vi "IMAQdx_set_attrib.vi"(4 "error in":errorcluster, 5 "value":variant, 6 "attribute":string, 7 "IMAQdx in":T1) -> (0 "error out":errorcluster, 2 "attrib out":variant, 3 "IMAQdx out":T1)   [LabVIEW 2010]
uses:
  <vilib>/userDefined/High Color/IMAQdx.ctl
  resource/objmgr/imaqdx.rc
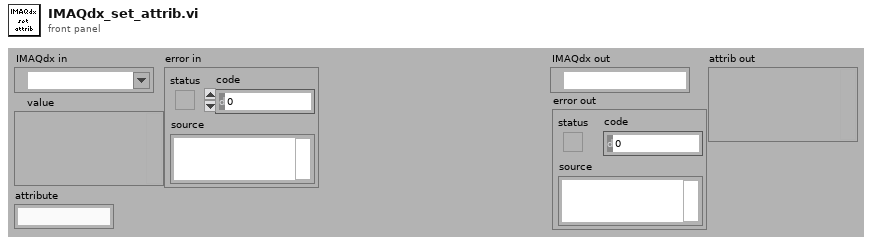
[diagram p1: front panel]
types:
  T1 = typedef "IMAQdx.ctl" = refnum<k21>
  T2 = typedef "Type Descriptor Enumeration__ogtk.ctl" = enum8{"<Null>", "I8", "I16", "I32", "I64", "U8", "U16", "U32", "U64", "SGL", "DBL", "EXT", "CSG", "CDB", "CXT", "0x0F", "0x10", "0x11", "0x12", "0x13", "0x14", "Enum U8", "Enum U16", "Enum U32", "Enum U64", "SGL PQ", "DBL PQ", "EXT PQ", "CSG PQ", "CDB PQ", "CXT PQ", "0x1F", "0x20", "Boolean", "0x22", "0x23", "0x24", "0x25", "0x26", "0x27", "0x28", "0x29", "0x2A", "0x2B", "0x2C", "0x2D", "0x2E", "0x2F", "String", "0x31", "Path", "Pict", "0x34", "0x35", "0x36", "DAQ", "0x38", "0x39", "0x3A", "0x3B", "0x3C", "0x3D", "0x3E", "0x3F", "Array", "0x41", "0x42", "0x43", "0x44", "0x45", "0x46", "0x47", "0x48", "0x49", "0x4A", "0x4B", "0x4C", "0x4D", "0x4E", "0x4F", "Cluster", "0x51", "0x52", "Variant", "Waveform", "0x55", "0x56", "0x57", "0x58", "0x59", "0x5A", "0x5B", "0x5C", "0x5D", "0x5E", "0x5F", "0x60", "0x61", "0x62", "0x63", "0x64", "0x65", "0x66", "0x67", "0x68", "0x69", "0x6A", "0x6B", "0x6C", "0x6D", "0x6E", "0x6F", "Refnum"}
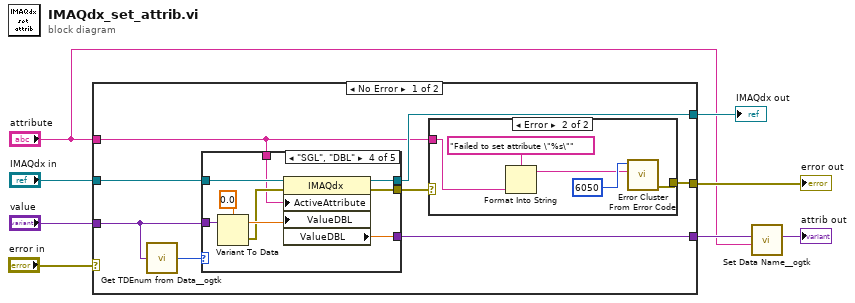
[diagram p0: block diagram]
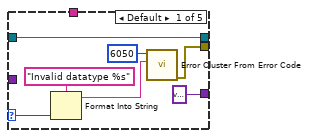
[diagram p3: hidden frame]
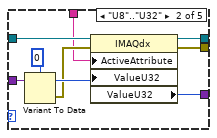
[diagram p4: hidden frame]
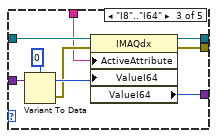
[diagram p5: hidden frame]
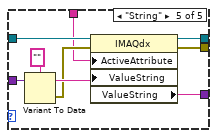
[diagram p6: hidden frame]
diagram:
  n1 = case shown="No Error" "error in" {
    selector: "error in" -> [_ w67]
    tunnel: [w16 w66] -> w8
    tunnel: "IMAQdx in" -> [w15 w66]
    tunnel: "value" -> [w9 w65]
    tunnel: "attribute" -> [w11 _]
    tunnel: [w12 w67] -> w6
    tunnel: [w10 w65] -> w4
    frame No Error {
      n2 = call <userlib>:"Get TDEnum from Data__ogtk.vi"("Data"=w9) -> ("Type Descriptor Enumeration"=w14:T2)  [unwired: 4 in]
      n3 = case shown="\"SGL\", \"DBL\"" w14 {
        selector: w14 -> [w27 _ _ _ _]
        tunnel: [w28 w37 w46 w55 w64] -> w16
        tunnel: w15 -> [w28 w36 w45 w54 w63]
        tunnel: w9 -> [_ w33 w42 w51 w60]
        tunnel: w11 -> [_ w31 w40 w49 w58]
        tunnel: [w24 w30 w39 w48 w57] -> w13
        tunnel: [variant ("Variant") w29 w38 w47 w56] -> w10
        frame Default {
          n4 = Format Into String(format string="Invalid datatype %s", w27) -> (resulting string=w23:string)  [unwired: 2 in, 1 out]
          n5 = call <vilib>:"Error Cluster From Error Code.vi"("error message (\"\")"=w23, "error code (0)"=6050) -> ("error out"=w24:errorcluster)  [unwired: 7 in]
        }
        frame "U8".."U32" {
          n6 = Variant To Data(Variant=w33, type=u32 0 ("ValueU32")) -> (error out=w32:errorcluster, data=w35:u32)  [unwired: 1 in]
          n7 = property class="IMAQdx"(reference=w36, error in=w32, "ActiveAttribute"=w31, "ValueU32"=w35) -> (reference out=w37:T1, error out=w30:errorcluster, "ValueU32"=w29:u32)
        }
        frame "I8".."I64" {
          n8 = Variant To Data(Variant=w42, type=i64 0 ("ValueU32")) -> (error out=w41:errorcluster, data=w44:i64)  [unwired: 1 in]
          n9 = property class="IMAQdx"(reference=w45, error in=w41, "ActiveAttribute"=w40, "ValueI64"=w44) -> (reference out=w46:T1, error out=w39:errorcluster, "ValueI64"=w38:i64)
        }
        frame "SGL", "DBL" {
          n10 = Variant To Data(Variant=w51, type=0.0 ("ValueU32")) -> (error out=w50:errorcluster, data=w53:dbl)  [unwired: 1 in]
          n11 = property class="IMAQdx"(reference=w54, error in=w50, "ActiveAttribute"=w49, "ValueDBL"=w53) -> (reference out=w55:T1, error out=w48:errorcluster, "ValueDBL"=w47:dbl)
        }
        frame "String" {
          n12 = Variant To Data(Variant=w60, type="" ("ValueU32")) -> (error out=w59:errorcluster, data=w62:string)  [unwired: 1 in]
          n13 = property class="IMAQdx"(reference=w63, error in=w59, "ActiveAttribute"=w58, "ValueString"=w62) -> (reference out=w64:T1, error out=w57:errorcluster, "ValueString"=w56:string)
        }
      }
      n14 = case shown="Error" w13 {
        tunnel: w11 -> [_ w18]
        tunnel: [_ w17] -> w12
        frame No Error {
        }
        frame Error {
          n15 = Format Into String(format string="Failed to set attribute \"%s\"", w18) -> (resulting string=w19:string)  [unwired: 2 in, 1 out]
          n16 = call <vilib>:"Error Cluster From Error Code.vi"("error message (\"\")"=w19, "error code (0)"=6050) -> ("error out"=w17:errorcluster)  [unwired: 7 in]
        }
      }
    }
    frame Error {
    }
  }
  "IMAQdx out" <- w8
  "error out" <- w6
  n17 = call <userlib>:"Set Data Name__ogtk.vi"("Data Name"="attribute", "Data"=w4) -> ("Renamed Data"=→"attrib out":variant)  [unwired: 8 in, 1 out]
